vi "Get Version.vi"() -> ()   [LabVIEW 2013]
uses:
  SubVIs/States.ctl
panel:
  out "Version":string
  in  "stop":bool
  in  "Open":bool
  in  "LabVIEW Versions Available":u16(ring) items=["LabVIEW 8.5", "LabVIEW 8.6", "LabVIEW 2009", "LabVIEW 2010", "LabVIEW 2011"]
  in  "Use VI":bool
  in  "VI":path
  # "SCC Demo"
  # "v 2.1"
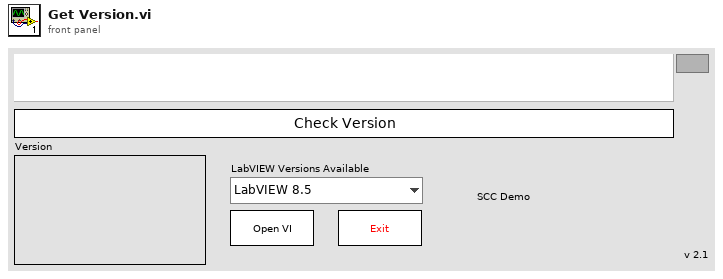
[diagram p1: front panel]
types:
  T1 = typedef "States.ctl" = enum16{"Get VI version", "Exit", "Open VI", "Wait on Command", "Determine VI", "Get LV Versions"}
  T2 = enum8{"Enabled", "Disabled", "Disabled and Grayed Out"}
  T3 = enum32{"invalid app kind", "Development System", "Run Time System", "Student Edition", "Embedded LabVIEW", "Evaluation", "Custom"}
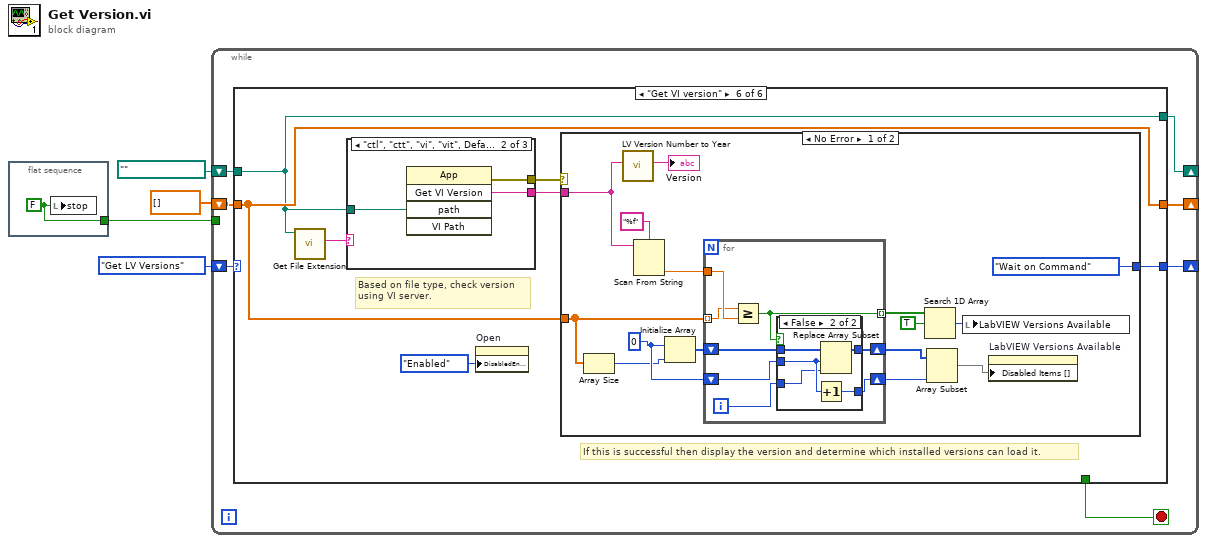
[diagram p0: block diagram]
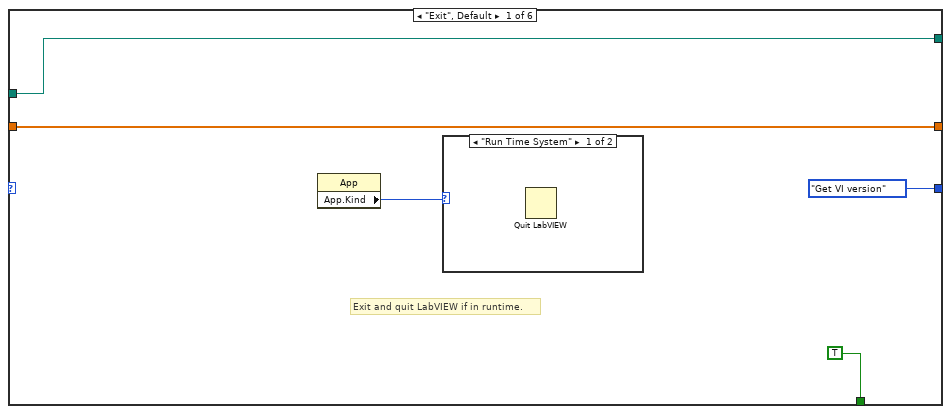
[diagram p2: hidden frame]
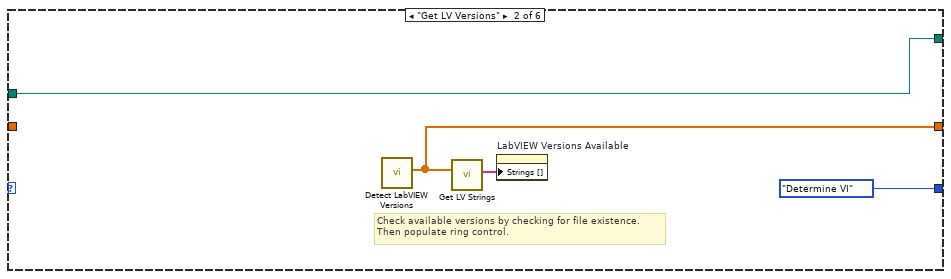
[diagram p4: hidden frame]
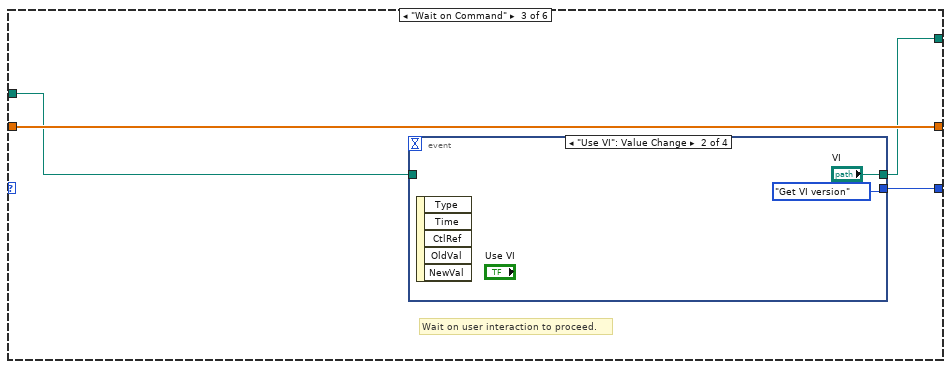
[diagram p5: hidden frame]
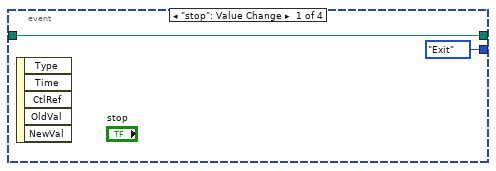
[diagram p6: hidden frame]
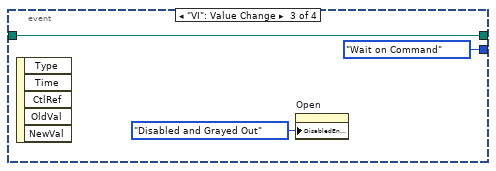
[diagram p7: hidden frame]
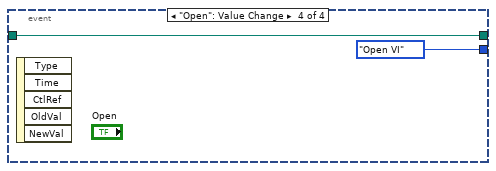
[diagram p8: hidden frame]
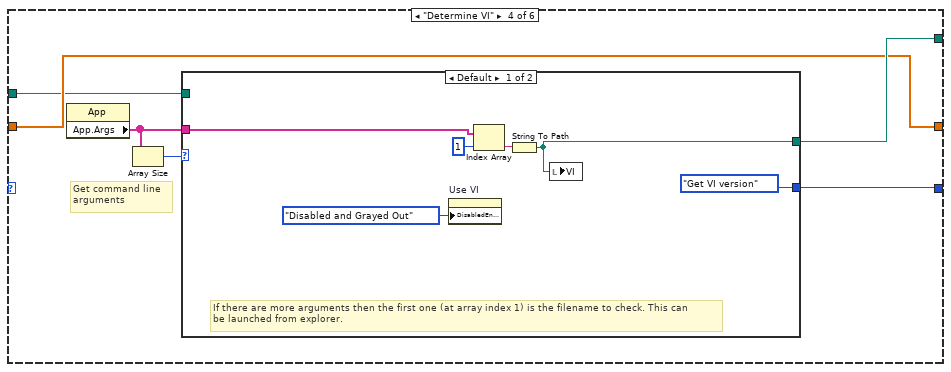
[diagram p9: hidden frame]
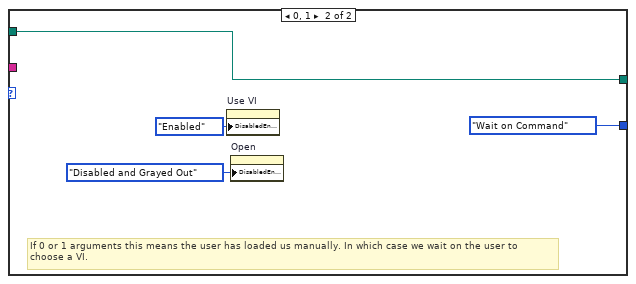
[diagram p10: hidden frame]
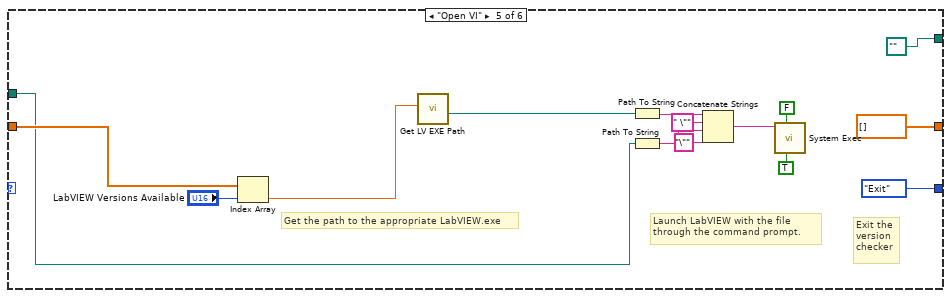
[diagram p11: hidden frame]
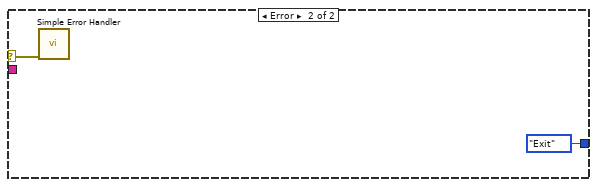
[diagram p13: hidden frame]
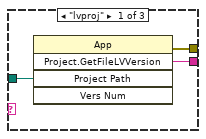
[diagram p14: hidden frame]
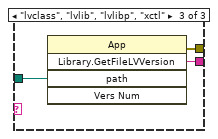
[diagram p15: hidden frame]
diagram:
  n1 = flat-sequence {
    tunnel: [w5] -> w1
    frame #0 {
      w5 = FALSE ("stop")
      n2 = local write "stop"(w5) -> ()
    }
  }
  n3 = while {
    shift-right: [w10] -> _
    shift-left: States."Get LV Versions" ("States") -> [w12]
    shift-right: [w11] -> _
    shift-left: dbl[] [] ("LabVIEW Versions") -> [w9]
    shift-right: [w8] -> _
    shift-left: path "" ("VI") -> [w7]
    tunnel: w1 -> [_]
    stop <- w6 stop-if-true
    n4 = case shown="\"Get VI version\"" w12 {
      tunnel: [w13 w20 w25 w37 dbl[] [] ("LabVIEW Versions") w70] -> w11
      tunnel: [States."Get VI version" ("States") States."Determine VI" ("States") w24 w35 States."Exit" ("States") w71] -> w10
      tunnel: w9 -> [w13 _ w25 w37 w65 w70]
      tunnel: [w14 w18 w22 w38 path "" ("VI") w69] -> w8
      tunnel: w7 -> [w14 w18 w23 w36 w62 w69]
      tunnel: [TRUE _ _ _ _ _] -> w6
      frame "Exit", Default {
        # "Exit and quit LabVIEW if in runtime."
        n5 = property class="App"() -> ("App.Kind"=w17:T3)  [unwired: 2 in, 2 out]
        n6 = case shown="\"Run Time System\"" w17 {
          frame "Run Time System" {
            n7 = Quit LabVIEW() -> ()  [unwired: 1 in]
          }
          frame "Development System", Default {
          }
        }
      }
      frame "Get LV Versions" {
        # "Check available versions by checking for file existence.\nThen populate ring control."
        n8 = call "Detect LabVIEW Versions.vi"() -> ("LabVIEW Versions"=w20:dbl[])  [unwired: 11 in]
        n9 = call "Get LV Strings.vi"("Versions"=w20) -> ("LabVIEW Strings"=w21:string[])  [unwired: 10 in]
        n10 = property on="LabVIEW Versions Available" class="Ring (strict)"("Strings []"=w21) -> ()  [unwired: 2 in, 2 out]
      }
      frame "Wait on Command" {
        # "Wait on user interaction to proceed."
        n11 = event shown="[1] \"Use VI\": Value Change" {
          selector: _ -> [_ _ _ _]
          dyn-events: _ -> [_ _ _ _]
          timeout: _ -> [_ _ _ _]
          tunnel: [States."Exit" ("States") States."Get VI version" ("States") States."Wait on Command" ("States") States."Open VI" ("States")] -> w24
          tunnel: w23 -> [w26 _ w32 w33]
          tunnel: [w26 "VI" w32 w33] -> w22
          event "stop": Value Change {
            n12 = event-data() -> ()  [unwired: 1 in, 5 out]
          }
          event "Use VI": Value Change {
            n13 = event-data() -> ()  [unwired: 1 in, 5 out]
          }
          event "VI": Value Change {
            n14 = event-data() -> ()  [unwired: 1 in, 5 out]
            n15 = property on="Open" class="Bool"("DisabledEnum"=T2."Disabled and Grayed Out" ("Disabled")) -> ()  [unwired: 2 in, 2 out]
          }
          event "Open": Value Change {
            n16 = event-data() -> ()  [unwired: 1 in, 5 out]
          }
        }
      }
      frame "Determine VI" {
        # "Get command line\narguments"
        n17 = property class="App"() -> ("App.Args"=w39:string[])  [unwired: 2 in, 2 out]
        n18 = Array Size(array=w39) -> (size(s)=w40:i32)
        n19 = case shown="Default" w40 {
          tunnel: [w45 w48] -> w38
          tunnel: w39 -> [w43 _]
          tunnel: w36 -> [_ w48]
          tunnel: [States."Get VI version" ("States") States."Wait on Command" ("t")] -> w35
          frame Default {
            # "If there are more arguments then the first one (at array index 1) is the filename to check. This can\nbe launched from explorer."
            n20 = property on="Use VI" class="Bool"("DisabledEnum"=T2."Disabled and Grayed Out" ("Disabled")) -> ()  [unwired: 2 in, 2 out]
            n21 = Index Array(array=w43, index=1) -> (element=w46:string)
            n22 = String To Path(string=w46) -> (path=w45:path)
            n23 = local write "VI"(w45) -> ()
          }
          frame 0, 1 {
            # "If 0 or 1 arguments this means the user has loaded us manually. In which case we wait on the user to\nchoose a VI."
            n24 = property on="Use VI" class="Bool"("DisabledEnum"=T2."Enabled" ("Disabled")) -> ()  [unwired: 2 in, 2 out]
            n25 = property on="Open" class="Bool"("DisabledEnum"=T2."Disabled and Grayed Out" ("Disabled")) -> ()  [unwired: 2 in, 2 out]
          }
        }
      }
      frame "Open VI" {
        # "Exit the \nversion \nchecker"
        # "Launch LabVIEW with the file\nthrough the command prompt."
        # "Get the path to the appropriate LabVIEW.exe"
        n26 = Index Array(array=w65, index="LabVIEW Versions Available") -> (element=w52:dbl)
        n27 = call "Get LV EXE Path.vi"("LabVIEW Version Number"=w52) -> ("appended path"=w51:path)  [unwired: 10 in]
        n28 = Path To String(path=w51) -> (string=w61:string)
        n29 = Path To String(path=w62) -> (string=w59:string)
        n30 = Concatenate Strings(w61, " \"" ("string"), w59, "\"" ("string")) -> (w58:string)
        n31 = call <vilib>:"System Exec.vi"("run minimized? (F)"=TRUE, "wait until completion? (T)"=FALSE, "command line"=w58) -> ()  [unwired: 5 in, 4 out]
      }
      frame "Get VI version" {
        # "If this is successful then display the version and determine which installed versions can load it."
        # "Based on file type, check version\nusing VI server."
        n32 = call <vilib>:"Get File Extension.vi"("file"=w69) -> ("lowercase file extension"=w66:string)  [unwired: 7 in, 3 out]
        n33 = case shown="\"ctl\", \"ctt\", \"vi\", \"vit\", Default" w66 {
          tunnel: [w106 w110 w113] -> w72
          tunnel: w69 -> [w107 w109 w112]
          tunnel: [w105 w108 w111] -> w68
          frame "lvproj" {
            n34 = invoke class="App" method="Project.GetFileLVVersion"("Project Path"=w107) -> (error out=w105:errorcluster, "Project.GetFileLVVersion"=w106:string)  [unwired: 4 in, 3 out]
          }
          frame "ctl", "ctt", "vi", "vit", Default {
            n35 = invoke class="App" method="Get VI Version"("path"=w109) -> (error out=w108:errorcluster, "GetVIVers"=w110:string)  [unwired: 4 in, 3 out]
          }
          frame "lvclass", "lvlib", "lvlibp", "xctl" {
            n36 = invoke class="App" method="Library.GetFileLVVersion"("path"=w112) -> (error out=w111:errorcluster, "Library.GetFileLVVersion"=w113:string)  [unwired: 4 in, 3 out]
          }
        }
        n37 = property on="Open" class="Bool"("DisabledEnum"=T2."Enabled" ("Disabled")) -> ()  [unwired: 2 in, 2 out]
        n38 = case shown="No Error" w68 {
          selector: w68 -> [_ w103]
          tunnel: w72 -> [w86 _]
          tunnel: [States."Wait on Command" ("States") States."Exit" ("States")] -> w71
          tunnel: w70 -> [w73 _]
          frame No Error {
            w78 = u16 0
            n39 = Array Size(array=w73) -> (size(s)=w76:i32)
            n40 = call "LV Version Number to Year.vi"("VI Version"=w86) -> ("LabVIEW Version"=→"Version":string)  [unwired: 10 in]
            n41 = Scan From String(format string="%f", input string=w86) -> (output 1=w75:dbl)  [unwired: 3 in, 3 out]
            n42 = Initialize Array(w78, w76) -> (w77:u16[])
            n43 = for {
              tunnel: w73 -> [w88] mode=indexing
              tunnel: w75 -> [w89]
              tunnel: [w92] -> w82 mode=indexing
              shift-right: [w94] -> w79
              shift-left: w77 -> [w95]
              shift-right: [w91] -> w80
              shift-left: w78 -> [w93]
              i -> [w90]
              n44 = Greater Or Equal?(x=w88, y=w89) -> (x >= y?=w92:bool)
              n45 = case shown="False" w92 {
                tunnel: w95 -> [w96 w102]
                tunnel: [w96 w101] -> w94
                tunnel: w93 -> [w97 w100]
                tunnel: [w97 w99] -> w91
                tunnel: w90 -> [_ w98]
                frame True {
                }
                frame False {
                  n46 = Increment(x=w100) -> (x+1=w99:u16)
                  n47 = Replace Array Subset(array=w102, new element=w98, index=w100) -> (w101:u16[])
                }
              }
            }
            n48 = Search 1D Array(1D array=w82, element=TRUE) -> (index of element=w84:i32)  [unwired: 1 in]
            n49 = Array Subset(array=w79, length=w80) -> (w81:u16[])  [unwired: 1 in]
            n50 = local write "LabVIEW Versions Available"(w84) -> ()
            n51 = property on="LabVIEW Versions Available" class="Ring (strict)"("Disabled Items []"=w81) -> ()  [unwired: 2 in, 2 out]
          }
          frame Error {
            n52 = call <vilib>:"Simple Error Handler.vi"("error in (no error)"=w103) -> ()  [unwired: 4 in, 5 out]
          }
        }
      }
    }
  }
